vi "Launcher - DMM HAL.vi"(6 "Worker Alias":string, 8 "error in":errorcluster, 9 "Initialization Data":T1, 11 "DMM HAL in":refnum<class "DMM HAL.lvclass">) -> (0 "error out":errorcluster)   [LabVIEW 2020]
doc: "This VI launches the Head Worker of a Workers application."
uses:
  Workers/Base Classes/DMM HAL/Initialization Data.ctl
  Workers/Base Classes/DMM HAL/Response Cases.ctl
  Workers/Base Classes/DMM HAL/DMM HAL.lvclass
  C:/Program Files (x86)/National Instruments/LabVIEW 2020/vi.lib/addons/_Workers/Library/Classes/Worker/Worker.lvclass
  <vilib>/addons/_Workers/Debugger/Debug Client/Debug Client.lvlib
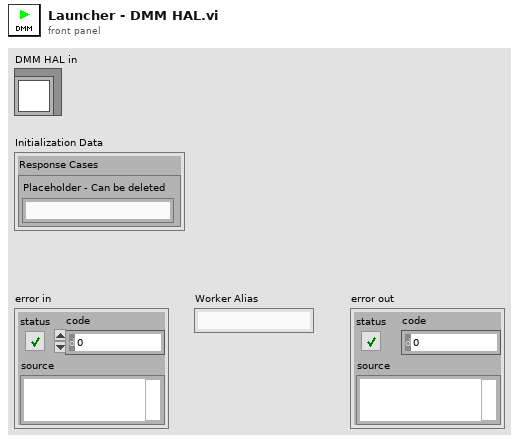
[diagram p1: front panel]
types:
  T1 = typedef "DMM HAL.lvclass/Initialization Data.ctl" = cluster{"Response Cases":T2}
  T2 = typedef "DMM HAL.lvclass/Response Cases.ctl" = cluster{"Placeholder - Can be deleted":string}
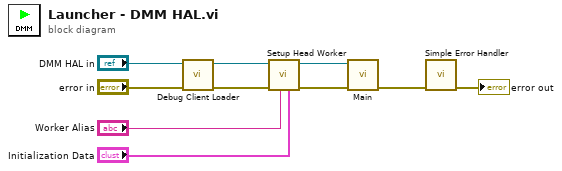
[diagram p0: block diagram]
diagram:
  n1 = call <vilib>:"Debug Client Loader.vi"("error in (no error)"="error in", "Worker"="DMM HAL in") -> ("error out"=w3:errorcluster, "Worker out"=w1:refnum<class "DMM HAL.lvclass">)  [unwired: 8 in]
  n2 = call-dynamic "Setup Head Worker.vi"("Initalization Data"="Initialization Data", "Worker Alias"="Worker Alias", "error in"=w3, "Worker"=w1) -> ("error out"=w10:errorcluster, "Worker out"=w7:refnum<class "DMM HAL.lvclass">)  [unwired: 6 in]
  n3 = call-dynamic "Main.vi"("Error in"=w10, "Worker"=w7) -> ("error out"=w8:errorcluster)  [unwired: 8 in, 1 out]
  n4 = call <vilib>:"Simple Error Handler.vi"("error in (no error)"=w8) -> ("error out"=→"error out":errorcluster)  [unwired: 4 in, 4 out]
